vi "模块配置读取.vi"(8 "error in (no error)":errorcluster caption="错误输入（无错误）") -> (0 "error out":errorcluster caption="错误输出")   [LabVIEW 2022 SP3, in "斯坦道CODcr.lvlib"]
uses:
  <vilib>/Utility/config.llb/NI_LVConfig.lvlib
  <userlib>/_OpenG.lib/variantconfig/variantconfig.llb/openg_variant_configuration_file.lvlib
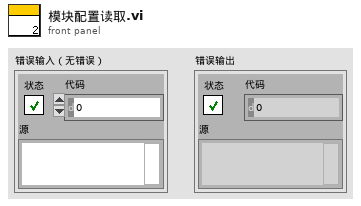
[diagram p1: front panel]
types:
  T1 = typedef "NI_LVConfig.lvlib/Config Data RefNum.ctl" = refnum<k1>
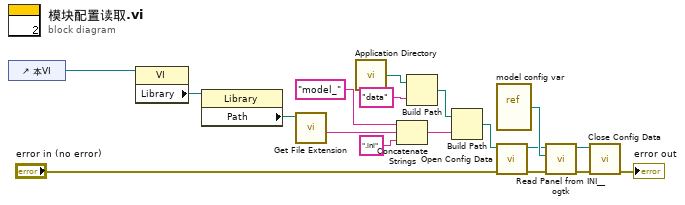
[diagram p0: block diagram]
diagram:
  n1 = control-ref of="本VI"() -> (w7:refnum<vi>)
  n2 = property class="VI"(reference=w7) -> ("Library"=w8:refnum<vi>)  [unwired: 1 in, 2 out]
  n3 = property class="Library"(reference=w8) -> ("Path"=w2:path)  [unwired: 1 in, 2 out]
  n4 = call <vilib>:"Get File Extension.vi"("file"=w2) -> ("filename without extension"=w1:string)  [unwired: 6 in, 4 out]
  n5 = call <vilib>:"Application Directory.vi"() -> ("Application Directory"=w10:path)
  n6 = Concatenate Strings("model_" ("字符串"), w1, ".ini" ("字符串")) -> (w6:string)
  n7 = Build Path(base path=w10, name or relative path="data" ("名称或相对路径")) -> (appended path=w9:path)
  n8 = Build Path(base path=w9, name or relative path=w6) -> (appended path=w3:path)
  n9 = vi-ref "model config var.vi"() -> (w15:refnum<vi>)
  n10 = call <vilib>:"Open Config Data.vi"("error in (no error)"="error in (no error)", "configuration file path"=w3) -> ("error out"=w17:errorcluster, "refnum"=w14:T1)  [unwired: 7 in, 1 out]
  n11 = call <userlib>:"Read Panel from INI__ogtk.vi"("error in (no error)"=w17, "VI ref"=w15, "refnum"=w14) -> ("error out"=w18:errorcluster, "refnum out"=w16:T1)  [unwired: 7 in]
  n12 = call <vilib>:"Close Config Data.vi"("error in (no error)"=w18, "refnum"=w16) -> ("error out"=→"error out":errorcluster)  [unwired: 8 in, 1 out]
